vi "Stop Core.vi"(10 "final error code":i32, 11 "Nested in":refnum<class "User Inteface.lvclass">) -> (3 "Nested out":refnum<class "User Inteface.lvclass">)   [LabVIEW 2020, in "User Inteface.lvlib" / "User Inteface.lvclass"]
doc: "(<B>Filename</B>: Actor Framework.lvlib:Actor.lvclass:Stop Core.vi)\n\nDefines what the actor does before it stops. Use the <B>final error code</B> input to determine whether the actor shut down in response to an error.\n\nBy default, this method does nothing. A descendant class may override it to define behavior, such as shutting down any processes the actor initiated in its override of the Actor Core method."
uses:
  User Inteface.lvclass
  <vilib>/ActorFramework/Actor/Actor.lvclass
  User Inteface.lvclass/User Inteface.ctl
  <vilib>/ActorFramework/Stop Msg/Stop Msg.lvclass
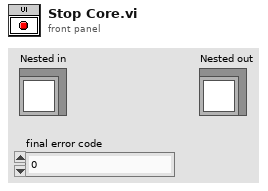
[diagram p1: front panel]
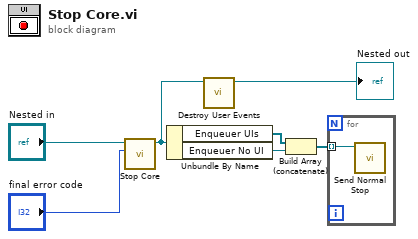
[diagram p0: block diagram]
diagram:
  n1 = call-parent "Stop Core.vi"("final error code"="final error code", "Actor in"="Nested in") -> ("Actor out"=w4:refnum<class "User Inteface.lvclass">)  [unwired: 9 in]
  n2 = Unbundle By Name(w4) -> ("Enqueuer UIs"=w3:refnum<class "Message Enqueuer.lvclass">[], "Enqueuer No UI"=w2:refnum<class "Message Enqueuer.lvclass">)
  n3 = call "Destroy User Events.vi"("UI Template in"=w4) -> ("UI Template out"=→"Nested out":refnum<class "User Inteface.lvclass">)  [unwired: 10 in]
  n4 = Build Array (concatenate)(w3, w2) -> (w1:refnum<class "Message Enqueuer.lvclass">[])
  n5 = for {
    tunnel: w1 -> [w8] mode=indexing
    n6 = call <vilib>:"Send Normal Stop.vi"("Message Enqueuer"=w8) -> ()  [unwired: 10 in, 1 out]
  }
